vi "SwissSPAD Live_SS3 Duty Cycle to Gate Parameters.vi"(6 "Period (ns)":dbl, 8 "Gate Definition Mode":T3, 9 "Reversed Shift":bool, 10 "Gate Width (ns)":dbl min=0.0 max=100.0, 11 "Gate Definition in":T1) -> (1 "Enabled State":T2(ring), 3 "Gate Definition out":T1)   [LabVIEW 2021]
uses:
  SwissSPAD Live_SS3 Gate Definition.ctl
  SS3 Gate Width Definition Mode.ctl
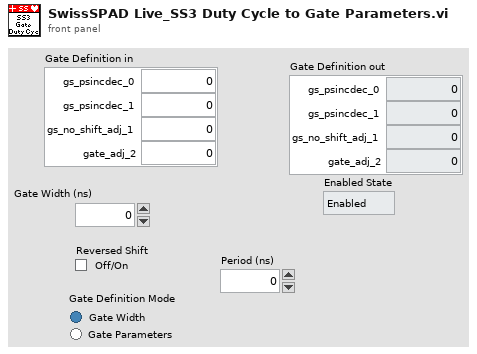
[diagram p1: front panel]
types:
  T1 = typedef "SwissSPAD Live_SS3 Gate Definition.ctl" = cluster{"gs_psincdec_0":u32, "gs_psincdec_1":u32, "gs_no_shift_adj_1":u32, "gate_adj_2":u32}
  T2 = enum8{"Enabled", "Disabled", "Disabled and Grayed Out"}
  T3 = typedef "SS3 Gate Width Definition Mode.ctl" = enum32{"Item 0", "Item 1"}
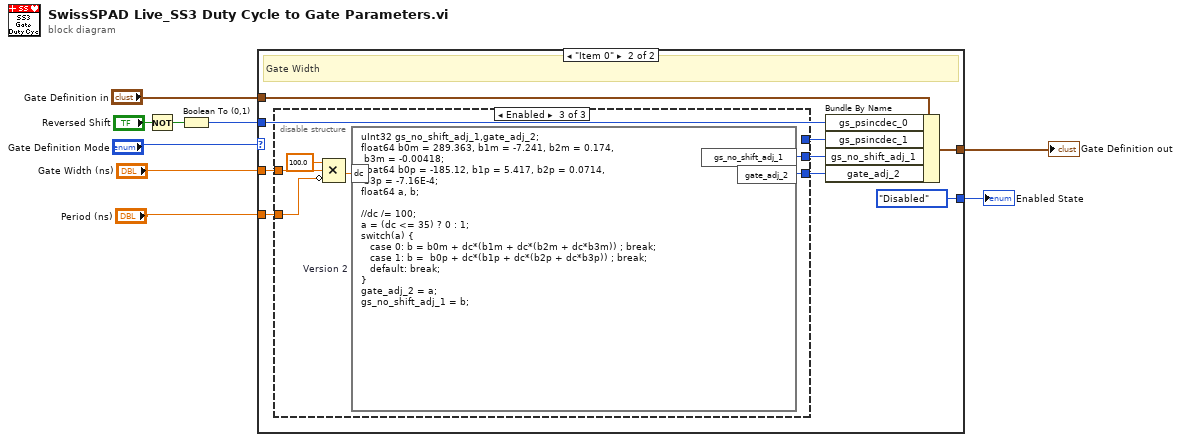
[diagram p0: block diagram]
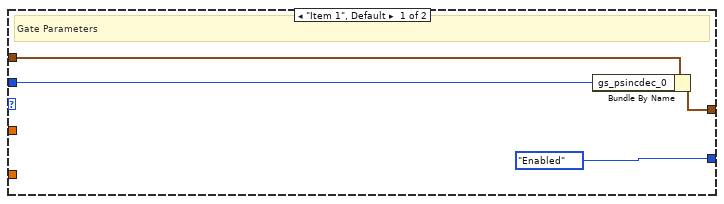
[diagram p2: hidden frame]
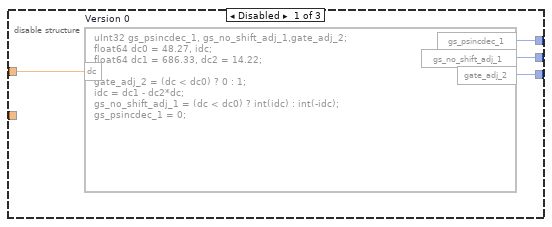
[diagram p3: hidden frame]
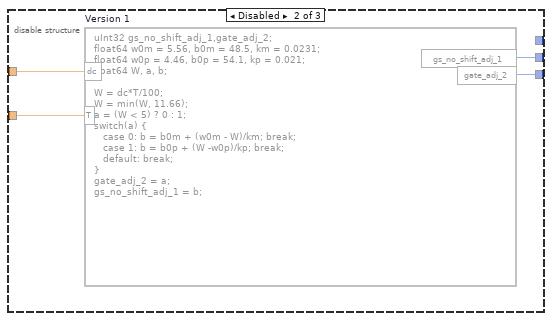
[diagram p4: hidden frame]
diagram:
  n1 = Not(x="Reversed Shift") -> (.not. x?=w7:bool)
  n2 = Boolean To (0,1)(Boolean=w7) -> (0, 1=w6:i16)
  n3 = case shown="\"Item 0\"" "Gate Definition Mode" {
    tunnel: [w13 w22] -> w9
    tunnel: w6 -> [w12 w21]
    tunnel: "Gate Width (ns)" -> [_ w20]
    tunnel: [T2."Enabled" ("Disabled") T2."Disabled" ("Disabled")] -> w3
    tunnel: "Gate Definition in" -> [w10 w15]
    tunnel: "Period (ns)" -> [_ w14]
    frame "Item 1", Default {
      # "Gate Parameters"
      n4 = Bundle By Name(cluster=w10, "gs_psincdec_0"=w12) -> (w13:T1)
    }
    frame "Item 0" {
      # "Gate Width"
      n5 = disable-structure shown="Enabled" {
        disable-tunnel: w20 -> [w26 w30 w36]
        disable-tunnel: [w25 _ _] -> w19
        disable-tunnel: [w24 w29 w35] -> w18
        disable-tunnel: [w23 w28 w34] -> w17
        disable-tunnel: w14 -> [_ w27 w32]
        frame Disabled {
          n6 = formula code="uInt32 gs_psincdec_1, gs_no_shift_adj_1,gate_adj_2;\nfloat64 dc0 = 48.27, idc;\nfloat64 dc1 = 686.33, dc2 = 14.22;\n\ngate_adj_2 = (dc < dc0) ? 0 : 1;\nidc = dc1 - dc2*dc;\ngs_no_shift_adj_1 = (dc < dc0) ? int(idc) : int(-idc);\ngs_psincdec_1 = 0;" "Version 0"("dc"=w26) -> ("gs_psincdec_1"=w25:u32, "gs_no_shift_adj_1"=w24:u32, "gate_adj_2"=w23:u32)
        }
        frame Disabled {
          n7 = formula code="uInt32 gs_no_shift_adj_1,gate_adj_2;\nfloat64 w0m = 5.56, b0m = 48.5, km = 0.0231;\nfloat64 w0p = 4.46, b0p = 54.1, kp = 0.021;\nfloat64 W, a, b;\n  \nW = dc*T/100;\nW = min(W, 11.66);\na = (W < 5) ? 0 : 1;\nswitch(a) {\n   case 0: b = b0m + (w0m - W)/km; break;\n   case 1: b = b0p + (W -w0p)/kp; break;\n   default: break;\n}\ngate_adj_2 = a;\ngs_no_shift_adj_1 = b;" "Version 1"("dc"=w30, "T"=w27) -> ("gs_no_shift_adj_1"=w29:u32, "gate_adj_2"=w28:u32)
        }
        frame Enabled {
          n8 = Compound Arithmetic op=MULTIPLY(100.0 ("value"), w36, invert w32) -> (w33:dbl)
          n9 = formula code="uInt32 gs_no_shift_adj_1,gate_adj_2;\nfloat64 b0m = 289.363, b1m = -7.241, b2m = 0.174,\n b3m = -0.00418;\nfloat64 b0p = -185.12, b1p = 5.417, b2p = 0.0714,\n b3p = -7.16E-4;\nfloat64 a, b;\n  \n//dc /= 100;\na = (dc <= 35) ? 0 : 1;\nswitch(a) { \n   case 0: b = b0m + dc*(b1m + dc*(b2m + dc*b3m)) ; break;\n   case 1: b =  b0p + dc*(b1p + dc*(b2p + dc*b3p)) ; break;\n   default: break;\n}\ngate_adj_2 = a;\ngs_no_shift_adj_1 = b;" "Version 2"("dc"=w33) -> ("gs_no_shift_adj_1"=w35:u32, "gate_adj_2"=w34:u32)
        }
      }
      n10 = Bundle By Name(cluster=w15, "gs_psincdec_0"=w21, "gs_psincdec_1"=w19, "gs_no_shift_adj_1"=w18, "gate_adj_2"=w17) -> (w22:T1)
    }
  }
  "Gate Definition out" <- w9
  "Enabled State" <- w3
